vi "Check Scaling.vi"(8 "error in (no error)":errorcluster, 11 "GenericGuiAO in":refnum<class "GenericGuiAO.lvclass">) -> (0 "error out":errorcluster, 3 "GenericGuiAO out":refnum<class "GenericGuiAO.lvclass">)   [LabVIEW 2020, in "VolatusDAQGenericGUI.lvlib" / "GenericGuiAO.lvclass"]
uses:
  GenericGuiAO.lvclass
  GenericGuiAO.lvclass/GenericGuiAO.ctl
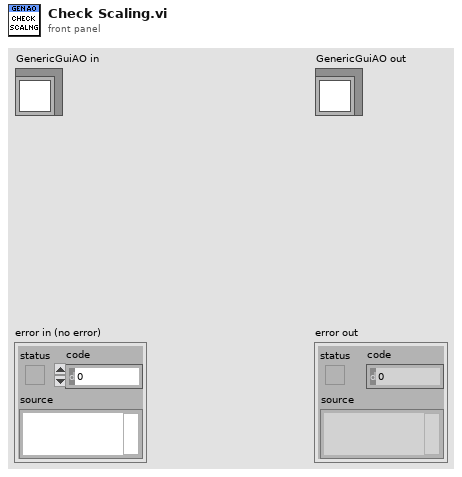
[diagram p1: front panel]
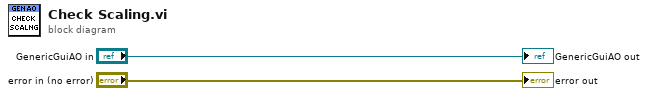
[diagram p0: block diagram]
diagram:
  "error out" <- "error in (no error)"
  "GenericGuiAO out" <- "GenericGuiAO in"
